vi "Read Param_I.vi"(8 "error in (no error)":errorcluster, 11 "Param in":T1) -> (0 "error out":errorcluster, 1 "PAR_sh":dbl[](array[numeric]), 2 "PAR_I":i32[](array[numeric]), 3 "Param out":T1)   [LabVIEW 2019, in "Inputs.lvlib"]
uses:
  Inputs.lvlib
  Ctl/Param.ctl
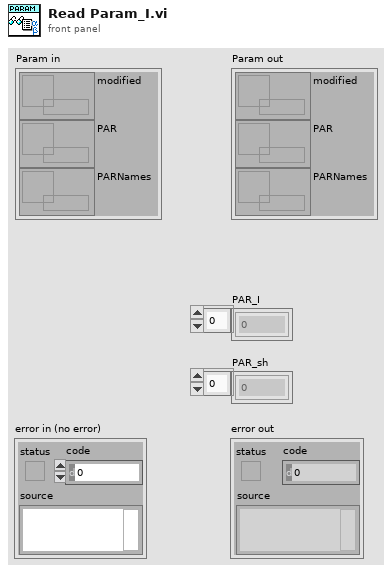
[diagram p1: front panel]
types:
  T1 = typedef "Inputs.lvlib/Param.ctl" = cluster{"modified":refnum<data-value>, "PAR":refnum<data-value>, "PARNames":refnum<data-value>}
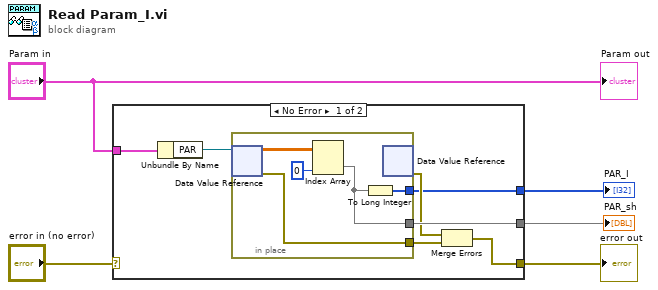
[diagram p0: block diagram]
diagram:
  n1 = case shown="No Error" "error in (no error)" {
    selector: "error in (no error)" -> [_ w18]
    tunnel: [w8 w18] -> w1
    tunnel: "Param in" -> [w7 _]
    tunnel: [w11 _] -> w2
    tunnel: [w6 _] -> w3
    frame No Error {
      n2 = Unbundle By Name(w7) -> ("PAR"=w12:refnum<data-value>)
      n3 = in-place {
        in-place-border: [w17] -> w10
        in-place-border: [w14] -> w11
        in-place-border: [w13] -> w6
        n4 = in-place-dvr #1(w12) -> (w16:dbl[][], w17:errorcluster)
        n5 = Index Array(array=w16, index (col)=0 ("disabled index (col)")) -> (element=w14:dbl[])  [unwired: 1 in]
        n6 = To Long Integer(number=w14) -> (32bit integer=w13:i32[])
        n7 = in-place-dvr #1() -> (w9:errorcluster)  [unwired: 1 in, 1 out]
      }
      n8 = Merge Errors(w9, w10) -> (w8:errorcluster)
    }
    frame Error {
    }
  }
  "error out" <- w1
  "PAR_I" <- w3
  "PAR_sh" <- w2
  "Param out" <- "Param in"
